vi "Get Temp Winding.vi"(8 "error in":errorcluster, 11 "HSU MCU V2 in":refnum<class "HSU MCU V2.lvclass">) -> (0 "error out":errorcluster, 2 "Temp Winding":dbl, 3 "HSU MCU V2 out":refnum<class "HSU MCU V2.lvclass">)   [LabVIEW 2024, in "HSU MCU V2.lvclass"]
uses:
  HSU MCU V2.lvclass
  HSU MCU V2.lvclass/HSU MCU V2.ctl
  DBCCommunication/DBC Communication.lvclass
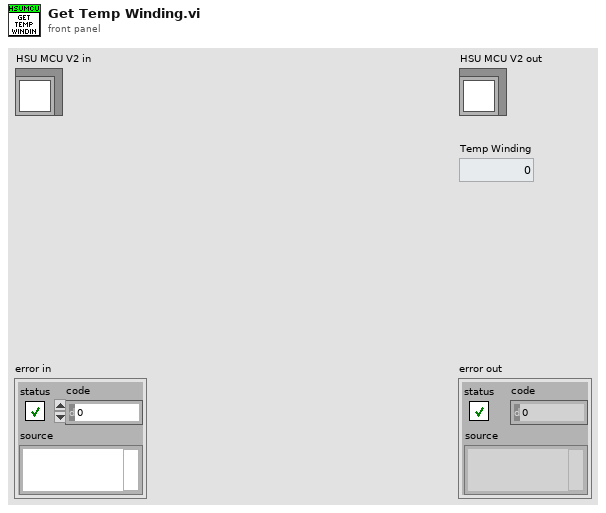
[diagram p1: front panel]
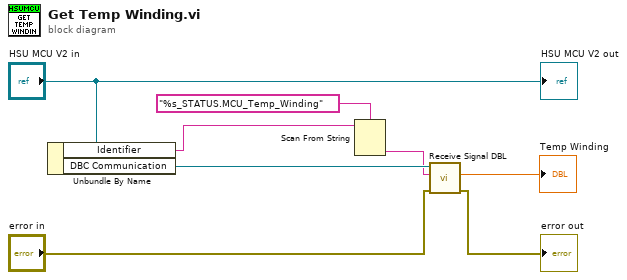
[diagram p0: block diagram]
diagram:
  n1 = Unbundle By Name("HSU MCU V2 in") -> ("Identifier"=w8:string, "DBC Communication"=w5:refnum<class "DBC Communication.lvclass">)
  n2 = Scan From String(format string="%s_STATUS.MCU_Temp_Winding", input string=w8) -> (output 1=w4:string)  [unwired: 3 in, 3 out]
  n3 = call "Receive Signal DBL.vi"("error in"="error in", "Signal Name"=w4, "DBC Communication in"=w5) -> ("error out"=→"error out":errorcluster, "Value"=→"Temp Winding":dbl)  [unwired: 6 in, 1 out]
  "HSU MCU V2 out" <- "HSU MCU V2 in"
